vi "BundleByName.vi"() -> ()   [LabVIEW 2021]
panel:
  out "Cluster":cluster{"String":string, "String 2":string}
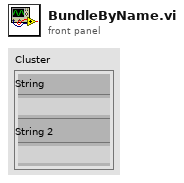
[diagram p1: front panel]
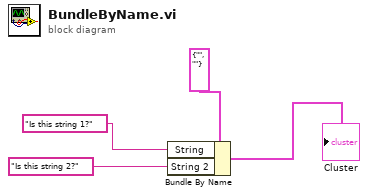
[diagram p0: block diagram]
diagram:
  n1 = Bundle By Name "Bundle By Name"(cluster=cluster{"String":string, "String 2":string} {"String"="", "String 2"=""} ("Cluster"), "String"="Is this string 1?", "String 2"="Is this string 2?") -> (→"Cluster":cluster{"String":string, "String 2":string})
